vi "OpenALPR-base.vi"(9 "image path to recognise":path, 10 "Max Possibility":i32=3, 11 "Default Country":string="hu") -> (1 "Processed Recognise Data:":string[][](array[string]), 2 "Detected Licence Plates as String":string, 3 "Init Return":string)   [LabVIEW 2014]
doc: "This project is help to integrate the OpnelALPR open source ALPR system to LabVIEW (for LV 2014 or newer versions). Everything is documented in the LV and C++ codes, if you want to find more information about the project, what this readme contains. The project also contains a html help for the example LW program, which could be find in the Help directory in the project.\n\n<b>Important!!!</b>\nThe „openalpr_32” directory contains the 2.3 version of the OpnelALPR open source ALPR system. For the sucesfull operation please copy the „openalpr_32” directory to C:/ in a folder (or whether you want). And create a \"OPENALPR_PATH\" environment variable, which have to point to the directory which contains the \"openalpr_32\" directory. The environment variable’s value must be the path of the directory, which contains the „openalpr_32” directory, not the „openalpr_32” directory’s path itself. (eg. “C:\\OpenALPR\\alpr_32”, where the “OPENALPR_PATH” environment variable’s value is “C:\\OpenALPR”)"
uses:
  OpenALPR_LabVIEW/OpenALPR in LabView.lvlib
panel:
  out "Place of the Image":string
  # "Recognise:"
  # "Initialize:"
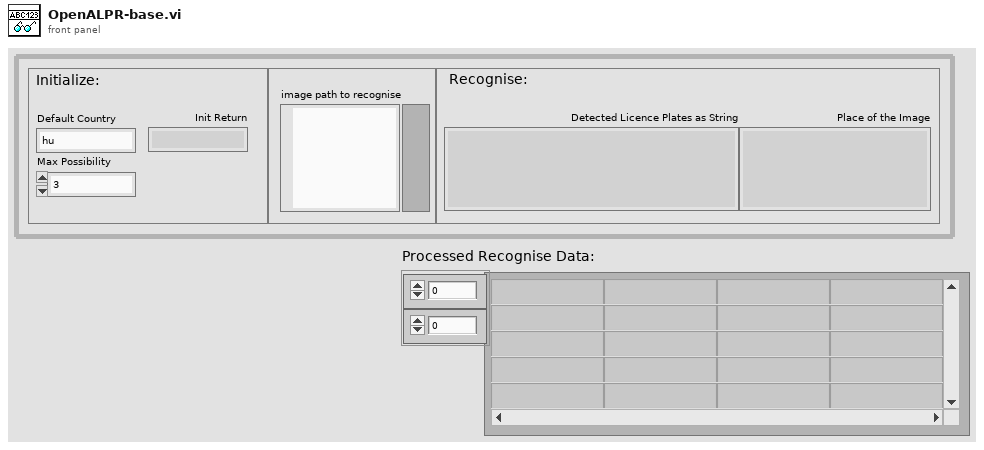
[diagram p1: front panel]
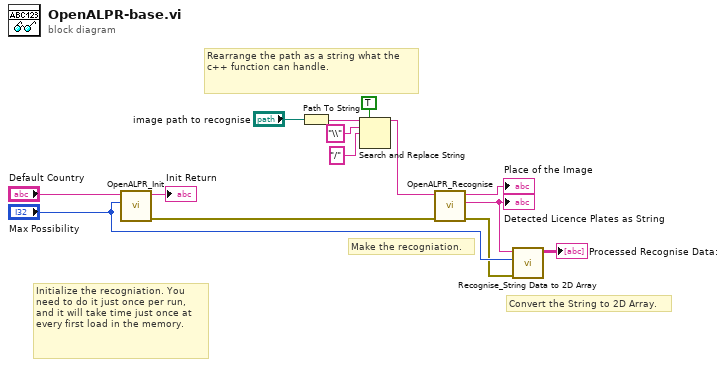
[diagram p0: block diagram]
diagram:
  # "Convert the String to 2D Array."
  # "Make the recogniation."
  # "Rearrange the path as a string what the c++ function can handle."
  # "Initialize the recogniation. You need to do it just once per run, and it will take time just once at every first load in the memory."
  n1 = call "OpenALPR_Init.vi"("Max possibility"="Max Possibility", "Default Country"="Default Country") -> ("error out"=w5:errorcluster, "Error"=→"Init Return":string)  [unwired: 8 in]
  n2 = Path To String(path="image path to recognise") -> (string=w11:string)
  n3 = Search and Replace String(replace all?=TRUE ("replace all? (F)"), input string=w11, search string="\\", replace string="/" ("replace string (\"\")")) -> (result string=w1:string)  [unwired: 4 in, 3 out]
  n4 = call "OpenALPR_Recognise.vi"("error in (no error)"=w5, "img"=w1) -> ("error out"=w4:errorcluster, "Detected plates"=w3:string, "img out"=→"Place of the Image":string)  [unwired: 7 in]
  "Detected Licence Plates as String" <- w3
  n5 = call "Recognise_String Data to 2D Array.vi"("error in (no error)"=w4, "Max Possibility"="Max Possibility", "Detected Licence Plates as String"=w3) -> ("Processed Recognise Data"=→"Processed Recognise Data:":string[][])  [unwired: 7 in, 1 out]
